vi "Test.vi"   [LabVIEW 2019]
doc: "This VI is only used for reporting robot status in the FRC 4265 architecture. Users should never enter Test mode via the FRC Driver Station. Instead, they should use the actuator testing interlock interface on the FRC 4265 Dashboard."
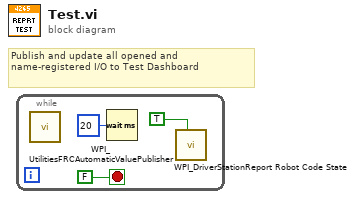
[diagram p0: block diagram]
diagram:
  # "Publish and update all opened and\nname-registered I/O to Test Dashboard"
  n1 = while {
    stop <- FALSE stop-if-true
    n2 = call <vilib>:"WPI_UtilitiesFRCAutomaticValuePublisher.vi"() -> ()  [unwired: 12 in]
    n3 = Wait (ms)(milliseconds to wait=u32 20) -> ()  [unwired: 1 out]
    n4 = call <vilib>:"WPI_DriverStationReport Robot Code State.vi"("Test"=TRUE ("Autonomous")) -> ()  [unwired: 10 in, 1 out]
  }
